vi "ReleaseRobot.vi"(0 "Universal Robot.lvclass in":refnum<class "Universal Robot.lvclass">, 5 "error in (no error)":errorcluster) -> (14 "Universal Robot.lvclass out":refnum<class "Universal Robot.lvclass">, 19 "error out":errorcluster)   [LabVIEW 2019, in "Universal Robot.lvclass"]
uses:
  Universal Robot.lvclass
  Universal Robot.lvclass/Universal Robot.ctl
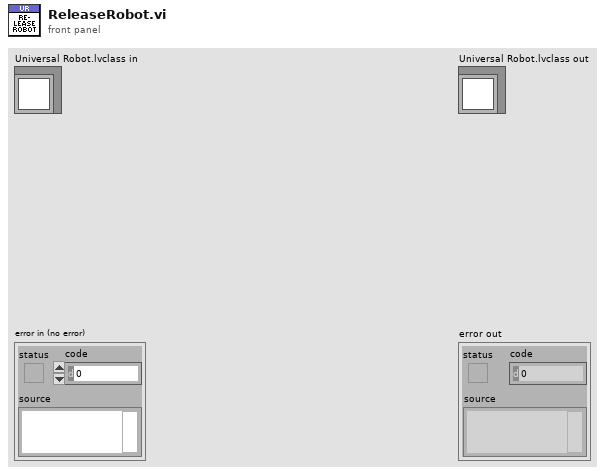
[diagram p1: front panel]
types:
  T1 = typedef "Semaphore RefNum" = refnum<k1>
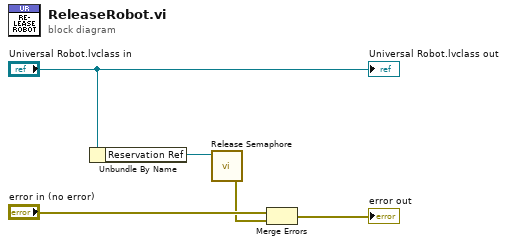
[diagram p0: block diagram]
diagram:
  n1 = Unbundle By Name("Universal Robot.lvclass in") -> ("Reservation Ref"=w5:T1)
  n2 = call <vilib>:"Release Semaphore.vi"("semaphore"=w5) -> ("error out"=w2:errorcluster)  [unwired: 5 in, 1 out]
  n3 = Merge Errors("error in (no error)", w2) -> (→"error out":errorcluster)
  "Universal Robot.lvclass out" <- "Universal Robot.lvclass in"
